vi "LOAD CELL READ.vi"(8 "error in (no error)":errorcluster, 11 "main ref":T1) -> (0 "error out":errorcluster)   [LabVIEW 2025]
uses:
  controls/LAB-IQ UI Data.ctl
  Traction Loop/Traction Receipe Enum.ctl
  <vilib>/Analysis/baseanly.llb/Mean (DBL).vi
  <vilib>/Analysis/5stat.llb/RMS (DBL).vi
  <vilib>/Analysis/NI_AALBase.lvlib
  <vilib>/ptbypt/NI_PtbyPt.lvlib
  <vilib>/Analysis/NI_AALPro.lvlib
  <vilib>/Analysis/Matrix/NI_Matrix.lvlib
  <vilib>/Analysis/Matrix/Numeric/Conversions/Matrix To Array - RM.vi
  <vilib>/Analysis/Matrix/Numeric/Conversions/Array To Matrix - RA.vi
panel:
  out "Fload 3":dbl
  out "Fload 2":dbl
  out "Fload":dbl
  out "Friction":dbl
  out "Load Temp":dbl
  out "Zload":dbl
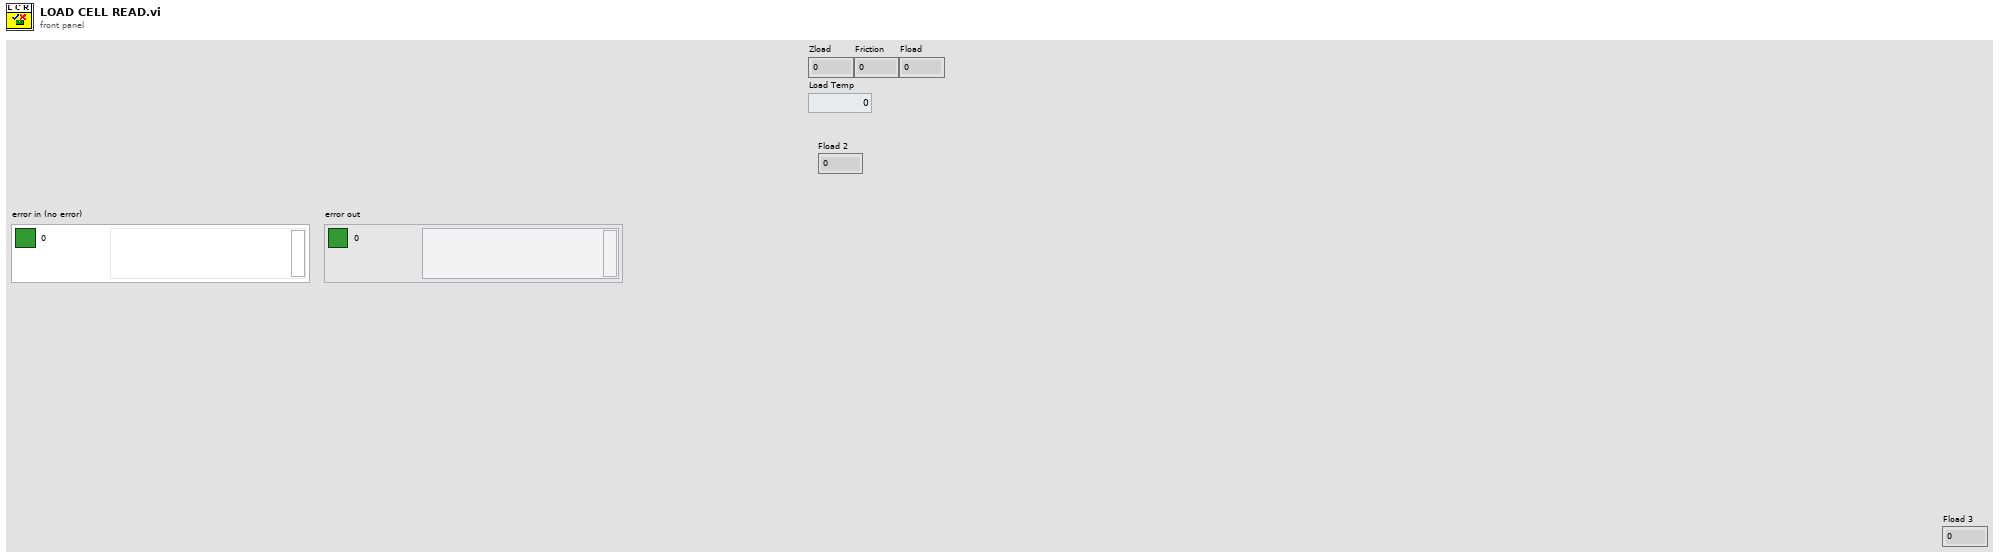
[diagram p1: front panel]
types:
  T1 = typedef "LAB-IQ UI Data.ctl" = cluster{"Main Home Screen":cluster{"GUI":refnum<vi>, "Platform Settings":refnum<vi>, "Configure":refnum<vi>, "Home":refnum<vi>, "EXIT":refnum<vi>, "service 2":refnum<vi>, "MainPage":refnum<vi>, "Analysis":refnum<vi>}, "Platform Settings":cluster{"mm/s  Surge":refnum<vi>, "Update Surge Speed":refnum<vi>, "Drive Error":refnum<vi>, "Disable Axis Jog Soft Limits":refnum<vi>, "mm/s  Sway":refnum<vi>, "Sway and Surge COM Status":refnum<vi>, "Heave COM Status":refnum<vi>, "Enable Platform":refnum<vi>, "Surge Forward Main":refnum<vi>, "Sway Right Main":refnum<vi>, "Sway Left Main":refnum<vi>, "Heave Down Main":refnum<vi>, "Heave Up main":refnum<vi>, "Update Sway Speed":refnum<vi>, "Update Heave Speed":refnum<vi>, "mm/s Heave":refnum<vi>, "mm/sec":refnum<vi>, "mm":refnum<vi>, "Surge Backward Main":refnum<vi>}, "Analysis Screen":cluster{"Analysis Home":refnum<vi>, "Surface Analysis":refnum<vi>, "Imaging":refnum<vi>, "Image Analysis":refnum<vi>, "Post Analysis":refnum<vi>}, "Config Screen":cluster{"Select Load Head":refnum<vi>, "Notes :":refnum<vi>, "FILE":refnum<vi>, "Sample ID :":refnum<vi>, "Operator ID :":refnum<vi>, "Operator Name :":refnum<vi>, "Auto":refnum<vi>}, "Motion Module":cluster{"zNL":refnum<vi>, "NL disp":refnum<vi>, "Rotary Tab":refnum<vi>, "Motion Direction:  3":refnum<vi>, "E.Velocity 2":refnum<vi>, "e.v/ssr 2":refnum<vi>, "Enter Fixed E.Velocity 2":refnum<vi>, "Enter Final SRR 2":refnum<vi>, "Enter initial SRR 2":refnum<vi>, "Enter Fixed SRR 2":refnum<vi>, "Enter the Final E.Velocity (m/s) 2":refnum<vi>, "Enter initial E.Velocity (m/s) 2":refnum<vi>, "Final Speed (RPM) 3":refnum<vi>, "Initial Speed (RPM) 2":refnum<vi>, "Enter the Final Velocity (m/s) 3":refnum<vi>, "Enter initial Velocity (m/s)  3":refnum<vi>, "Ramp Up 2":refnum<vi>, "TEST SELECTION":refnum<vi>, "SPEED SELECTION : ":refnum<vi>, "Angular Oscillation Set":refnum<vi>, "Traction":refnum<vi>, "Step Speed":refnum<vi>, "StepTable For Load-Speed":refnum<vi>, "StepTable For Speed":refnum<vi>, "Surge Forward MM":refnum<vi>, "Surge Backward MM":refnum<vi>, "M3 Image":refnum<vi>, "String 39":refnum<vi>, "Sway Left MM":refnum<vi>, "Sway Right MM":refnum<vi>, "Disable Axis Jog Soft Limits":refnum<vi>, "mm":refnum<vi>, "Heave Down MM":refnum<vi>, "Heave Up MM":refnum<vi>, "Wear Track Diameter (mm)":refnum<vi>, "Set WTD":refnum<vi>, "HomeScratch":refnum<vi>, "HomeRot":refnum<vi>, "PlaceModule":refnum<vi>, "Enter the Angle (Deg)":refnum<vi>, "Enter the Frequency (Hz)":refnum<vi>, "Motion Mode:":refnum<vi>, "LR Sway":refnum<vi>, "Rot Hor":refnum<vi>, "Scratch":refnum<vi>, "LR Cam":refnum<vi>, "MMBack":refnum<vi>, "MMNext":refnum<vi>, "Rot Ver":refnum<vi>, "Rotary Module Selection":refnum<vi>, "calculate rotary":refnum<vi>, "SPEED SELECTION : rotary":refnum<vi>, "Import 2":refnum<vi>, "Save 2":refnum<vi>, "File Path :  2":refnum<vi>, "String 45":refnum<vi>, "StepTable For Speed 3":refnum<vi>, "Enter the Speed(mm/sec)":refnum<vi>, "Enter the Speed(RPM)":refnum<vi>, "Enter Scratch Speed (mm/s):":refnum<vi>, "SwaySpeed Set":refnum<vi>, "Scartch Offset":refnum<vi>, "Motion type:":refnum<vi>, "HomeScratch 2":refnum<vi>, "Enter Scratch length (mm):":refnum<vi>, "Wear Track Diameter":refnum<vi>, "Rotary Speed Exced":refnum<vi>, "Scratch Mode":refnum<vi>, "No of Scratch":refnum<vi>}, "Environmental control":cluster{"Humidity  Status  3":refnum<vi>, "Low Temp  Status  2":refnum<vi>, "TK4 status 2":refnum<vi>, "Stage Temperature":refnum<vi>, "Sample Temperature":refnum<vi>, "Humidity (Amb)":refnum<vi>, "Clear List":refnum<vi>, "Add to list":refnum<vi>, "Wear":refnum<vi>, "Vibration":refnum<vi>, "Humidity (Chamber)":refnum<vi>, "Temperature (Chamber)":refnum<vi>, "ECR ":refnum<vi>, "Temperature (Amb)":refnum<vi>, "Microphone":refnum<vi>, "Acoustic Emission 3":refnum<vi>, "SNext":refnum<vi>, "APBack":refnum<vi>, "Enter the Temperature (°C):":refnum<vi>, "Enter the Stage \nTemperature (°C):":refnum<vi>, "Enter the Humidity (%Rh):":refnum<vi>, "Low Temp":refnum<vi>, "High Temp":refnum<vi>, "Humidity":refnum<vi>, "Sensors Picked":refnum<vi>}, "About Screen":cluster{"Password":refnum<vi>, "Home Service":refnum<vi>, "Advanced Setting":refnum<vi>, "About Tab":refnum<vi>, "ECR Port:":refnum<vi>, "Ramp Port:":refnum<vi>, "Installation/Replacement completed":refnum<vi>, "Loahead":refnum<vi>, "Heave and Surge COM Port:":refnum<vi>, "Sway COM Port:":refnum<vi>, "Temp Modbus:":refnum<vi>, "Humidity Port:":refnum<vi>, "Edit Gain Constants":refnum<vi>, "Save Gain Constants":refnum<vi>}, "Main Screen":cluster{"Main Screen Tab":refnum<vi>, "Angle and Frequency":refnum<vi>, "Stroke (mm)":refnum<vi>, "Angle (Deg)":refnum<vi>, "Main Speed Tab":refnum<vi>, "MTM MOTOR DISPLAY":refnum<vi>, "Disc Speed (m/sec)":refnum<vi>, "Ball Speed (m/sec)":refnum<vi>, "Disc Speed (RPM)":refnum<vi>, "Ball Speed (RPM)":refnum<vi>, "SPEED TAB":refnum<vi>, "Speed (m/sec)":refnum<vi>, "Set Speed (m/sec)":refnum<vi>, "Speed (RPM)":refnum<vi>, "Set Speed":refnum<vi>, "Time Tab":refnum<vi>, "Time ( HH:MM:SS ) 2":refnum<vi>, "Test Duration":refnum<vi>, "Test Duration 4":refnum<vi>, "TEST CYCLE":refnum<vi>, "TOTAL CYCLES":refnum<vi>, "Set Load (N)":refnum<vi>, "Temp Tabs":refnum<vi>, "Heater":refnum<vi>, "TK4 status":refnum<vi>, "ChamberTemp":refnum<vi>, "SetTmp":refnum<vi>, "Controller  Status":refnum<vi>, "ChamberTemp 2":refnum<vi>, "SetTmp 2":refnum<vi>, "Controller  Status 2":refnum<vi>, "ChamberTemp 3":refnum<vi>, "SetTmp 3":refnum<vi>, "Cooling":refnum<vi>, "Load Communication":refnum<vi>, "Ambient \nTemperature":refnum<vi>, "HumCOMStatus":refnum<vi>, "Ambient\n Humidity":refnum<vi>, "Freq (Hz)":refnum<vi>, "Load En":refnum<vi>, "NLt":refnum<vi>, "zNL 2":refnum<vi>, "Humidity On":refnum<vi>, "humidity disp":refnum<vi>, "Set Humidity":refnum<vi>, "NL disp 2":refnum<vi>, "Humidity On 2":refnum<vi>, "humidity disp 2":refnum<vi>, "Set Humidity 2":refnum<vi>, "NL disp 3":refnum<vi>, "AppLoadSeq scratch":refnum<vi>, "Stop Scratch":refnum<vi>, "ClrLog":refnum<vi>, "Trip Log":refnum<vi>, "STOP":refnum<vi>, "Start Test":refnum<vi>, "Test status":refnum<vi>, "AR Led":refnum<vi>, "Data":refnum<vi>, "Health":refnum<vi>, "Sway COM Status":refnum<vi>, "Heave COM Status":refnum<vi>, "Grp Tab":refnum<vi>, "Sub Graph":refnum<vi>, "SD (mm)":refnum<vi>, "Siliding distance Reset Graph":refnum<vi>, "SDGp":refnum<vi>, "Humidity Reset Graph":refnum<vi>, "HumrGp":refnum<vi>, "Acoustic Emission (mV)":refnum<vi>, "Aqucostic Reset Graph":refnum<vi>, "gACQUOS":refnum<vi>, "ECR RESET":refnum<vi>, "ECR":refnum<vi>, "Temperature Reset":refnum<vi>, "Acoustic Emission (mV) 2":refnum<vi>, "Aqucostic Reset Graph 2":refnum<vi>, "gACQUOS 2":refnum<vi>, "ECR RESET 2":refnum<vi>, "ECR 2":refnum<vi>, "Temperature Reset 2":refnum<vi>, "Temperature (deg c)":refnum<vi>, "Speed Reset Graph":refnum<vi>, "Speed Tab":refnum<vi>, "MTM DISC  SPEED":refnum<vi>, "MTM BALL SPEED":refnum<vi>, "speed mm/sec":refnum<vi>, "Hymidity":refnum<vi>, "Humidity Disable trip":refnum<vi>, "CoF Trip  2":refnum<vi>, "Depth Trip":refnum<vi>, "Weart Deapth":refnum<vi>, "Depth Reset Graph":refnum<vi>, "Weart":refnum<vi>, "Depthz":refnum<vi>, "Depth (µm)":refnum<vi>, "WearGp":refnum<vi>, "NL Trip 2":refnum<vi>, "Load pid":refnum<vi>, "Load Disable Trip":refnum<vi>, "Load Reset Graph":refnum<vi>, "NL Display 4":refnum<vi>, "Main Chart 3":refnum<vi>, "BACK":refnum<vi>, "Depth Trip 2":refnum<vi>, "COF TRIP ":refnum<vi>, "Friction Force (N)":refnum<vi>, "FF Reset Graph":refnum<vi>, "FF Disable Trip":refnum<vi>, "FF TRIP":refnum<vi>, "COF Disable Trip":refnum<vi>, "COF Reset Graph":refnum<vi>, "Start Test Temp":refnum<vi>, "zFF":refnum<vi>, "Friction Force (N) Graph":refnum<vi>, "Coefficient of Friction":refnum<vi>, "Scratch Start Test":refnum<vi>, "FF Tab":refnum<vi>, "Cyclic Friction Force (N)":refnum<vi>, "CZ FF":refnum<vi>, "Cyclic Friction Force (N) Graph":refnum<vi>, "Cyclic Coefficient of Friction":refnum<vi>, "Cyclic FF TRIP":refnum<vi>, "Cyclic FF Disable Trip":refnum<vi>, "cyclic COF Disable Trip":refnum<vi>, "cyclic COF TRIP":refnum<vi>, "cyclic COF Reset Graph":refnum<vi>, "Cyclic FF Reset Graph":refnum<vi>, "Test Trip":refnum<vi>, "Multi Scratch Pass":refnum<vi>, "Scratch Start Recording":refnum<vi>}, "Loading":cluster{"Indentation":refnum<vi>, "Reference Sample":refnum<vi>, "Load Cell Communication Slide":refnum<vi>, "com 3":refnum<vi>, "com":refnum<vi>, "DecaForce COM Status":refnum<vi>, "Update":refnum<vi>, "Clear 3":refnum<vi>, "seq":refnum<vi>, "Stribeck table":refnum<vi>, "Stribeck Table  For loading":refnum<vi>, "Loading Mode":refnum<vi>, "Enter the Final Load (N)":refnum<vi>, "Enter the CoF Trip":refnum<vi>, "Enter the Friction Force Trip":refnum<vi>, "Enter the Normal load Trip":refnum<vi>, "Enter the Load  (N)":refnum<vi>, "KiloForce":refnum<vi>, "DecaForce ":refnum<vi>, "MicroForce":refnum<vi>, "LHBack":refnum<vi>, "LHNext":refnum<vi>, "Enter the Loading Rate (N/min)":refnum<vi>, "Message":refnum<vi>, "Warning 2":refnum<vi>, "SSP 0.75":refnum<vi>, "SSP 0.5":refnum<vi>, "SSP 0.3":refnum<vi>, "Warning":refnum<vi>, "gui GIF":refnum<vi>, "Communication is established":refnum<vi>, "AppLoad 4":refnum<vi>, "Multipoint":refnum<vi>, "Load Selection":refnum<vi>}, "PID":cluster{"Ramp MulFac":refnum<vi>, "pulses LoadDiffRamp(2..10)":refnum<vi>, "PulseControlRamp(diff<=3N)":refnum<vi>, "SetLoadDeadband(%) Load(0-10N)":refnum<vi>, "PID gains out delay (microForce)":refnum<vi>, "Ramp":refnum<vi>, "Gain 2":refnum<vi>, "pulses LoadDiff(2..10)":refnum<vi>, "pulses LoadDiff(11..50)":refnum<vi>, "PulseControl(diff<=3N)":refnum<vi>, "SetLoadDeadband(%)  2":refnum<vi>, "Dummy Run":refnum<vi>, "Vertical load (N)":refnum<vi>, "AutoTune":refnum<vi>, "Offset 3 ":refnum<vi>, "apply load":refnum<vi>, "Offset  3":refnum<vi>, "apply load 2":refnum<vi>, "Enter ByPass Load":refnum<vi>, "reinit 3":refnum<vi>, "output range delay":refnum<vi>, "PID gains out delay":refnum<vi>, "Bypass Load":refnum<vi>, "pulsesSent":refnum<vi>, "pulses ":refnum<vi>, "actpid":refnum<vi>, "gFF Rot":refnum<vi>, "pulses LoadDiff(21..1000)":refnum<vi>, "Delay":refnum<vi>, "deadband":refnum<vi>}, "Config Parameters":cluster{"Tab Control 3":refnum<vi>, "Tab Control 19":refnum<vi>, "SAMPLES":refnum<vi>, "Re-initilaize":refnum<vi>, "Filter ON/OFF":refnum<vi>, "TracHomeSurgeOffsetCounts 10MM":refnum<vi>, "TracHomeSwayOffsetCounts 10MM":refnum<vi>, "Acoustic Emission:":refnum<vi>, "Apply Filter (FF)":refnum<vi>, "Filter% 2":refnum<vi>, "Apply Filter (Load)":refnum<vi>, "Filter% ":refnum<vi>, "Sway distance (mm)":refnum<vi>, "Surge distance (mm)":refnum<vi>, "DataSavingLoopDelay(ms)":refnum<vi>, "SAVE 2":refnum<vi>, "Enter Distance":refnum<vi>, "Sway Counts:":refnum<vi>, "Distance (mm): 3":refnum<vi>, "Surge Counts:":refnum<vi>, "Distance (mm): 2":refnum<vi>, "Distance (mm):":refnum<vi>, "Heave Counts:":refnum<vi>, "LRMHomeSurgeOffsetCounts":refnum<vi>, "LRMHomeSwayOffsetCounts":refnum<vi>, "TracHomeSurgeOffsetCounts 20MM":refnum<vi>, "TracHomeSwayOffsetCounts 20MM":refnum<vi>, "RotHomeSwayOffsetCounts":refnum<vi>, "RotHomeSurgeOffsetCounts":refnum<vi>, "Heave distance":refnum<vi>, "Zmm":refnum<vi>, "Heave Pulses/mm":refnum<vi>, "Surge Pulses/mm":refnum<vi>, "Sway Pulses/mm":refnum<vi>, "Heave Pitch":refnum<vi>, "Surge Pitch":refnum<vi>, "Sway Pitch":refnum<vi>, "Heave PPR":refnum<vi>, "Surge PPR":refnum<vi>, "Sway PPR":refnum<vi>, "Tab Control 5":refnum<vi>, "Tab Control 14":refnum<vi>, "Tab Control 26":refnum<vi>, "AE":refnum<vi>, "Heave Loop Delay":refnum<vi>, "Heave PID Speed":refnum<vi>, "Surge Jog Speed":refnum<vi>, "Heave Jog Speed":refnum<vi>, "Sway Loop Delay":refnum<vi>, "Sway PID Speed":refnum<vi>, "Sway Jog Speed":refnum<vi>, "DEPTH TRIP VALUE":refnum<vi>, "LOAD TRIP VALUE":refnum<vi>, "DEPTH TRIP   ENABLE":refnum<vi>, "LOAD TRIP  ENABLE":refnum<vi>, "CYCLIC FF TRIP VALUE":refnum<vi>, "FF TRIP VALUE":refnum<vi>, "CYCLIC CoF TRIP VALUE":refnum<vi>, "COF TRIP VALUE":refnum<vi>, "CYCLIC COF TRIP  ENABLE":refnum<vi>, "CYCLIC FF TRIP  ENABLE":refnum<vi>, "FF TRIP  ENABLE":refnum<vi>, "COF TRIP  ENABLE":refnum<vi>, "JOG TRIP LOAD VALUE (N)":refnum<vi>, "Rotary Vertical":refnum<vi>, "Traction":refnum<vi>, "Scratch":refnum<vi>, "LRM CAM":refnum<vi>, "Sway LRM":refnum<vi>, "Rotary Horizontal":refnum<vi>}, "Loading Com Port":cluster{"ClearAll":refnum<vi>, "Mz(Nm)":refnum<vi>, "My(Nm)":refnum<vi>, "Mx(Nm)":refnum<vi>, "Save Dwell":refnum<vi>, "Acq Delay (ms)":refnum<vi>, "Burst Delay (ms)":refnum<vi>, "model":refnum<vi>, "SN":refnum<vi>, "FFx(N)":refnum<vi>, "Sensor IP":refnum<vi>, "Port":refnum<vi>, "FFy(N)":refnum<vi>, "Load(N)":refnum<vi>, "delete Handle":refnum<vi>, "Create Handle":refnum<vi>, "ft_data":refnum<vi>, "ft_range":refnum<vi>, "ft_data 2":refnum<vi>, "stop 6":refnum<vi>, "running_flag":refnum<vi>, "ft_udp_handle":refnum<vi>, "get-data-return":refnum<vi>, "get-range-return":refnum<vi>, "zero-return":refnum<vi>, "filter-return":refnum<vi>, "initial-return":refnum<vi>, "deleteHandle-result":refnum<vi>, "Load Cell Temp":refnum<vi>, "Load Cell":refnum<vi>, "ZeroAll":refnum<vi>, "FORCE (N)":refnum<vi>, "TORQUE (N-m)":refnum<vi>}, "Heave AND Surge":cluster{"SURGE POSE":refnum<vi>, "error out Read":refnum<vi>, "HEAVE POSE":refnum<vi>, "State":refnum<vi>, "Homed":refnum<vi>, "Sequence ID":refnum<vi>, "error out Write":refnum<vi>, "faultCode":refnum<vi>, "Ack ID":refnum<vi>, "SPEED":refnum<vi>, "Distance":refnum<vi>, "Mode Command":refnum<vi>, "Heave and Surge Read":refnum<vi>, "Read Heave Temp":refnum<vi>, "Spare 15":refnum<vi>, "Spare 14":refnum<vi>, "Spare 13":refnum<vi>, "Spare 12":refnum<vi>, "Spare 11":refnum<vi>, "Spare 10":refnum<vi>, "Spare 9":refnum<vi>, "Spare 8":refnum<vi>, "Spare 7":refnum<vi>, "Spare 6":refnum<vi>, "Spare 5":refnum<vi>, "Spare 4":refnum<vi>, "Spare 2":refnum<vi>, "Spare 1":refnum<vi>, "Node Id":refnum<vi>, "Spare 3":refnum<vi>, "SPARE 4":refnum<vi>, "SPARE 3":refnum<vi>, "SPARE 2":refnum<vi>, "SPARE 1":refnum<vi>, "fwMajor":refnum<vi>, "fwMinor":refnum<vi>, "Manual Write":refnum<vi>, "Heave and Surge Write":refnum<vi>, "SPARE 5":refnum<vi>, "Reserved ":refnum<vi>, "SPARE 8":refnum<vi>, "SPARE 6":refnum<vi>, "SPARE 7":refnum<vi>, "SPARE 17":refnum<vi>, "SPARE 16":refnum<vi>, "SPARE 15":refnum<vi>, "SPARE 14":refnum<vi>, "SPARE 13":refnum<vi>, "SPARE 12":refnum<vi>, "SPARE 11":refnum<vi>, "SPARE 10":refnum<vi>, "SPARE 9":refnum<vi>, "System UPTIME":refnum<vi>, "Missed Packets":refnum<vi>, "faultCode Surge Right":refnum<vi>, "faultCode Surge Left":refnum<vi>, "faultCode Heave":refnum<vi>, "UPLINK HEAVE":refnum<vi>, "DOWNLINK HEAVE":refnum<vi>}, "New PID LOGIC":cluster{"Fine Tune Zone":refnum<vi>, "PID SDelay":refnum<vi>, "Max_pos_limit":refnum<vi>, "Min_pos_limit":refnum<vi>, "i_limit":refnum<vi>, "pct_scale":refnum<vi>, "Deadband":refnum<vi>, "Kd":refnum<vi>, "Ki":refnum<vi>, "Kp":refnum<vi>, "Current Position":refnum<vi>, "Set Load":refnum<vi>, "Current Load":refnum<vi>, "Pulse delta":refnum<vi>, "Init Step":refnum<vi>, "Max Step Linit":refnum<vi>, "min_deadband_floor":refnum<vi>, "dynamic_spindle_noise_scalar":refnum<vi>, "min_finetune_floor":refnum<vi>, "filter_alpha":refnum<vi>, "PID":refnum<vi>}, "SWAY ":cluster{"fwMajor":refnum<vi>, "Homed":refnum<vi>, "Rotary POSE":refnum<vi>, "State":refnum<vi>, "SWAY POSE":refnum<vi>, "Ack ID":refnum<vi>, "faultCode":refnum<vi>, "Node Id":refnum<vi>, "fwMinor":refnum<vi>, "Spare 6":refnum<vi>, "Spare 5":refnum<vi>, "Spare 4":refnum<vi>, "Spare 3":refnum<vi>, "Spare 2":refnum<vi>, "Spare 1":refnum<vi>, "Spare 7":refnum<vi>, "SPARE  5":refnum<vi>, "error out Write  SWAY ":refnum<vi>, "error out Read SWAY ":refnum<vi>, "Manual Write SWAY ":refnum<vi>, "SWAY WRITE":refnum<vi>, "SPARE  4":refnum<vi>, "SPARE  3":refnum<vi>, "SPARE 2":refnum<vi>, "SPARE 1":refnum<vi>, "Spare 15":refnum<vi>, "Spare 14":refnum<vi>, "Spare 13":refnum<vi>, "Spare 12":refnum<vi>, "Spare 11":refnum<vi>, "Spare 9":refnum<vi>, "Spare 8":refnum<vi>, "SPEED":refnum<vi>, "Distance":refnum<vi>, "Mode Command":refnum<vi>, "Sequence ID":refnum<vi>, "SWAY READ":refnum<vi>, "Spare 10":refnum<vi>, "Read SWAY Temp":refnum<vi>, "faultCode Sway ":refnum<vi>, "Missed Packets":refnum<vi>, "System UPTIME sway":refnum<vi>, "SPARE 6":refnum<vi>, "SPARE 7":refnum<vi>, "SPARE 9":refnum<vi>, "SPARE 11":refnum<vi>, "SPARE 10":refnum<vi>, "SPARE 8":refnum<vi>, "SPARE 13":refnum<vi>, "SPARE 12":refnum<vi>, "SPARE 17":refnum<vi>, "SPARE 16":refnum<vi>, "SPARE 15":refnum<vi>, "SPARE 14":refnum<vi>, "Reserved":refnum<vi>, "faultCode Rotary":refnum<vi>, "UPLINK SWAY":refnum<vi>, "DOWNLINK SWAY":refnum<vi>}, "Analysis Screen":cluster{"Analysis Home":refnum<vi>, "Refresh 2":refnum<vi>, "MEAN 4":refnum<vi>, "SD 4":refnum<vi>, "VARIANCE 4":refnum<vi>, "MEAN  3":refnum<vi>, "SD  3":refnum<vi>, "VARIANCE  3":refnum<vi>, "MEAN 2":refnum<vi>, "SD  2":refnum<vi>, "VARIANCE 2":refnum<vi>, "MEAN":refnum<vi>, "SD":refnum<vi>, "VARIANCE":refnum<vi>, "File 4 Discription":refnum<vi>, "OPEN 4":refnum<vi>, "File Name 4":refnum<vi>, "OPEN 3":refnum<vi>, "File 3 Discription":refnum<vi>, "File Name 3":refnum<vi>, "Y-AXIS":refnum<vi>, "X-AXIS":refnum<vi>, "XY Graph":refnum<vi>, "File Name 2":refnum<vi>, "File Name 1":refnum<vi>, "OPEN 2":refnum<vi>, "OPEN 1":refnum<vi>, "File 1 Discription ":refnum<vi>, "File 2 Discription":refnum<vi>, "Export":refnum<vi>, "File Format":refnum<vi>}, "Traction":cluster{"faultCode Traction 2":refnum<vi>, "faultCode Traction 1":refnum<vi>, "Missed Packets":refnum<vi>, "System UPTIME Traction":refnum<vi>, "SPARE 17":refnum<vi>, "SPARE 16":refnum<vi>, "SPARE 15":refnum<vi>, "SPARE 14":refnum<vi>, "SPARE 13":refnum<vi>, "SPARE 12":refnum<vi>, "SPARE 11":refnum<vi>, "SPARE 10":refnum<vi>, "SPARE 9":refnum<vi>, "SPARE 8":refnum<vi>, "SPARE 7":refnum<vi>, "SPARE 6":refnum<vi>, "Reserved":refnum<vi>, "SPARE  5":refnum<vi>, "Manual Write TRACTION":refnum<vi>, "TRACTION WRITE":refnum<vi>, "SPARE  4":refnum<vi>, "SPARE  3":refnum<vi>, "SPARE 2":refnum<vi>, "SPARE 1":refnum<vi>, "Spare 7":refnum<vi>, "Spare 6":refnum<vi>, "Spare 5":refnum<vi>, "Spare 4":refnum<vi>, "Spare 2":refnum<vi>, "Spare 1":refnum<vi>, "Node Id":refnum<vi>, "Read TRACTION Temp":refnum<vi>, "fwMinor":refnum<vi>, "fwMajor":refnum<vi>, "faultCode":refnum<vi>, "TRACTION POSE":refnum<vi>, "TRACTION POSE 2":refnum<vi>, "Homed":refnum<vi>, "State":refnum<vi>, "Ack ID":refnum<vi>, "SPEED":refnum<vi>, "Distance":refnum<vi>, "Mode Command":refnum<vi>, "Sequence ID":refnum<vi>, "error out Read TRACTION":refnum<vi>, "error out Write  TRACTION":refnum<vi>, "TRACTION READ":refnum<vi>, "Spare 3":refnum<vi>, "Downlink traction":refnum<vi>, "Uplink Traction":refnum<vi>}, "Traction reciepe":cluster{"SRR Sweep Range (%) Stribeck":refnum<vi>, "Traction Receipe":refnum<vi>, "Total Execution Time":refnum<vi>, "Total Steps":refnum<vi>, "Duration / Step (s)  Stribeck":refnum<vi>, "STRIBECK Fixed SRR List (%)":refnum<vi>, "Duration / Step (s) Traction":refnum<vi>, "SRR Sweep Range (%) traction":refnum<vi>, "Rolling Speed (mm/s)":refnum<vi>, "Temperature Stages (°C)":refnum<vi>, "Ball Load (N)":refnum<vi>, "Lubricant Name":refnum<vi>, "Profile File Name":refnum<vi>, "SET entrainment Velocity":refnum<vi>, "Test Array Size":refnum<vi>, "SRR INDEX [ STRIBECK]":refnum<vi>, "Stribeck Size":refnum<vi>, "SET SRR":refnum<vi>, "ELAPSED TIMER ":refnum<vi>, "BALL SET RPM":refnum<vi>, "DISC SET RPM":refnum<vi>, "SET LOAD":refnum<vi>, "TEMPERATURE READ":refnum<vi>, "SET TEMPERATURE":refnum<vi>, "Traction Size":refnum<vi>, "DISC SPEED (rpm)":refnum<vi>, "BALL SPEED (rpm)":refnum<vi>, "BALL WEAR TRACK":refnum<vi>, "DISC WEARTRACK":refnum<vi>, "SRR INDEX [ TRACTION]":refnum<vi>, "Start Index Type":refnum<vi>, "Enum - Menu":refnum<vi>, "Ball (mm/sec)":refnum<vi>, "Disc (mm/sec)":refnum<vi>}, "Traction Control":cluster{"HomeTraction":refnum<vi>, "Demo Mode Display":refnum<vi>, "Traction Message":refnum<vi>, "Traction Step Update Details":refnum<vi>, "Main Tab sequence for selection":refnum<vi>, "Ramp Tab":refnum<vi>, "e.v/ssr":refnum<vi>, "Enter Fixed E.Velocity":refnum<vi>, "Enter Final SRR":refnum<vi>, "Enter initial SRR":refnum<vi>, "Enter Fixed SRR":refnum<vi>, "Enter the Final E.Velocity (m/s)":refnum<vi>, "Enter initial E.Velocity (m/s)":refnum<vi>, "Ball WTD":refnum<vi>, "E.Velocity":refnum<vi>, "Enter the Final Velocity (m/s)":refnum<vi>, "Enter initial Velocity (m/s)":refnum<vi>, "Ramp Up   Disc":refnum<vi>, "Initial DiscSpeed (RPM)":refnum<vi>, "Final Speed (RPM) Ball":refnum<vi>, "Final Speed (RPM)":refnum<vi>, "Initial Speed (RPM) Ball":refnum<vi>, "Enter the Final Velocity (m/s) Ball":refnum<vi>, "Enter initial Velocity (m/s) Ball":refnum<vi>, "Ramp Up":refnum<vi>, "ExceedBallSpeed step":refnum<vi>, "ExceedDiscSpeed":refnum<vi>, "BallSpeed Exceed Indication":refnum<vi>, "Apply":refnum<vi>, "SPEED SELECTION : MTM":refnum<vi>, "SPEED SELECTION : MTM 2":refnum<vi>, "TEST SELECTION (MTM)":refnum<vi>, "MTM Test Selection":refnum<vi>, "File Path Tab":refnum<vi>, "File Path String":refnum<vi>, "Save":refnum<vi>, "Save  2":refnum<vi>, "Import ":refnum<vi>, "File Path :":refnum<vi>, "Step Sequence Indication Tab":refnum<vi>, "Step Sequence Indication":refnum<vi>, "Calculate Step":refnum<vi>, "StepTable":refnum<vi>, "ExceedDiscSpeed  Cinstant Speed":refnum<vi>, "ExceedBallSpeed Constant":refnum<vi>, "TEST SELECTION (MTM) 2":refnum<vi>, "SPEED SELECTION : MTM 3":refnum<vi>, "MTM Test Selection 2":refnum<vi>, "Enter the Speed (m/sec): ":refnum<vi>, "Enter the Speed (m/sec):  2":refnum<vi>, "Enter the Speed (RPM):":refnum<vi>, "Lower Spped ":refnum<vi>, "Upper":refnum<vi>, "Enter the Speed (RPM):Ball":refnum<vi>, "Disc Motion Direction: ":refnum<vi>, "Ball Motion Direction :":refnum<vi>, "Motion Mode: ":refnum<vi>, "Wear Track Diameter (mm) ":refnum<vi>, "Disc Speed Indicator":refnum<vi>, "ExceedBallSpeed":refnum<vi>}, "Acquostic":cluster{"Last Config Rejected ":refnum<vi>, "rx command count":refnum<vi>, "Current Filter Id":refnum<vi>, "Isolated Gain":refnum<vi>, "DAQ Status":refnum<vi>, "error out":refnum<vi>, "error in (no error)":refnum<vi>, "Uplink Packet":refnum<vi>, "data out":refnum<vi>, "Downlink Packet":refnum<vi>, "Signal Energy":refnum<vi>, "Amplitude db_AE":refnum<vi>, "Peak Amplitude":refnum<vi>, "AE Ring-Down Counts":refnum<vi>, "Gains":refnum<vi>, "Manual Write Acquostic":refnum<vi>}}
  T2 = enum16{"INIT", "SETLOWPASSFILTER", "SETZERO", "GETSENSORINFO", "GETRANGE", "ZEROALL", "READDATA", "UNINITIAL", "DELETEHANDLE"}
  T3 = typedef "NI_Matrix.lvlib/RealMatrix.ctl" = dbl[][]
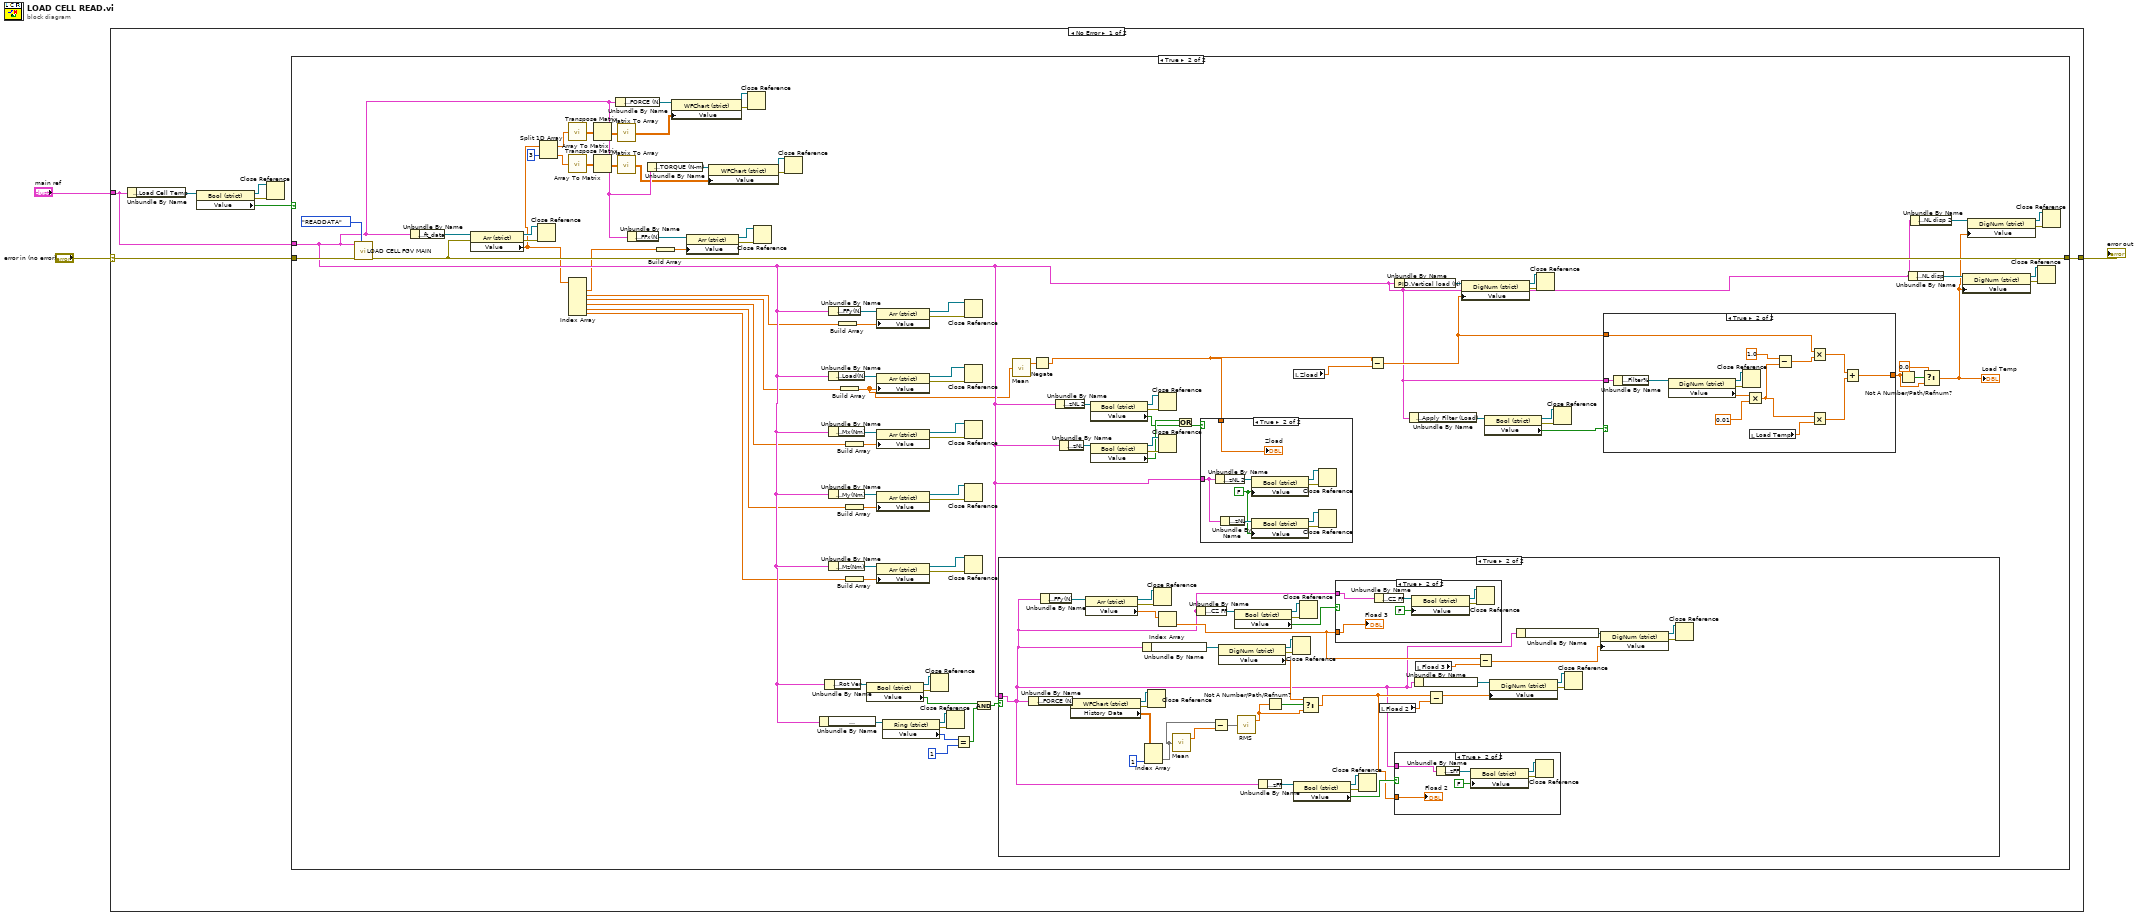
[diagram p0: block diagram]
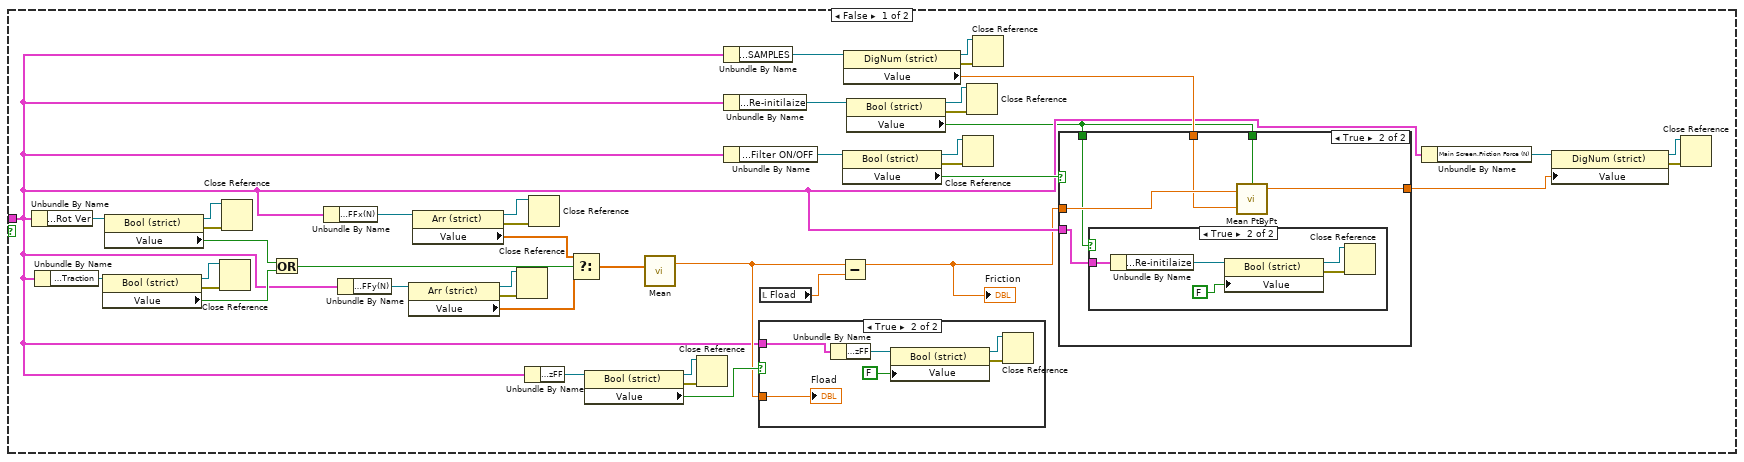
[diagram p3: hidden frame]
diagram:
  n1 = case shown="No Error" "error in (no error)" {
    selector: "error in (no error)" -> [w6 _]
    tunnel: "main ref" -> [w4 _]
    tunnel: [w5 _] -> w1
    frame No Error {
      n2 = Unbundle By Name(w4) -> ("Loading Com Port.Load Cell Temp"=w8:refnum<vi>)
      n3 = property class="Bool (strict)"(reference=w8) -> (reference out=w10:refnum<vi>, error out=w9:errorcluster, "Value"=w7:bool)  [unwired: 1 in]
      n4 = Close Reference(reference=w10, error in (no error)=w9) -> ()  [unwired: 1 out]
      n5 = case shown="True" w7 {
        tunnel: w6 -> [w11 w105]
        tunnel: [w11 w101] -> w5
        tunnel: w4 -> [_ w26]
        frame False {
        }
        frame True {
          n6 = call "LOAD CELL FGV MAIN.vi"("Enum"=T2."READDATA", "error in (no error)"=w105, "main ref"=w26) -> ("error IO"=w101:errorcluster)  [unwired: 8 in]
          n7 = Unbundle By Name(w26) -> ("Loading Com Port.ft_data"=w103:refnum<vi>)
          n8 = property class="Arr (strict)"(reference=w103, error in=w101) -> (reference out=w100:refnum<vi>, error out=w102:errorcluster, "Value"=w24:dbl[])
          n9 = Close Reference(reference=w100, error in (no error)=w102) -> ()  [unwired: 1 out]
          n10 = Split 1D Array(array=w24, index=3) -> (first subarray=w34:dbl[], second subarray=w31:dbl[])
          n11 = call-poly <vilib>:"Array To Matrix.vi"("Real 1D Array"=w34) -> ("Real Matrix (Column Vector)"=w36:T3)
          n12 = call-poly <vilib>:"Array To Matrix.vi"("Real 1D Array"=w31) -> ("Real Matrix (Column Vector)"=w33:T3)
          n13 = Index Array(array=w24) -> (element #1=w23:dbl, element #2=w21:dbl, element #3=w19:dbl, element #4=w18:dbl, element #5=w15:dbl, element #6=w13:dbl)  [unwired: 6 in]
          n14 = Transpose Matrix(1:w36) -> (0:w35:T3)
          n15 = Transpose Matrix(1:w33) -> (0:w32:T3)
          n16 = Unbundle By Name(w26) -> ("Loading Com Port.FORCE (N)"=w99:refnum<vi>)
          n17 = call-poly <vilib>:"Matrix To Array.vi"("Real Matrix"=w35) -> ("Real 2D Array"=w30:dbl[][])
          n18 = call-poly <vilib>:"Matrix To Array.vi"("Real Matrix"=w32) -> ("Real 2D Array"=w25:dbl[][])
          n19 = Unbundle By Name(w26) -> ("Loading Com Port.FFx(N)"=w94:refnum<vi>)
          n20 = Unbundle By Name(w26) -> ("Loading Com Port.TORQUE (N-m)"=w29:refnum<vi>)
          n21 = Build Array(w23) -> (w22:dbl[])
          n22 = property class="WFChart (strict)"(reference=w99, "Value"=w30) -> (reference out=w97:refnum<vi>, error out=w98:errorcluster)  [unwired: 1 in]
          n23 = property class="Arr (strict)"(reference=w94, "Value"=w22) -> (reference out=w96:refnum<vi>, error out=w95:errorcluster)  [unwired: 1 in]
          n24 = property class="WFChart (strict)"(reference=w29, "Value"=w25) -> (reference out=w27:refnum<vi>, error out=w28:errorcluster)  [unwired: 1 in]
          n25 = Close Reference(reference=w97, error in (no error)=w98) -> ()  [unwired: 1 out]
          n26 = Close Reference(reference=w96, error in (no error)=w95) -> ()  [unwired: 1 out]
          n27 = Close Reference(reference=w27, error in (no error)=w28) -> ()  [unwired: 1 out]
          n28 = Unbundle By Name(w26) -> ("Motion Module.Motion Mode:"=w43:refnum<vi>)
          n29 = Unbundle By Name(w26) -> ("Motion Module.Rot Ver"=w48:refnum<vi>)
          n30 = Unbundle By Name(w26) -> ("Loading Com Port.FFy(N)"=w91:refnum<vi>)
          n31 = Unbundle By Name(w26) -> ("Loading Com Port.Load(N)"=w90:refnum<vi>)
          n32 = Unbundle By Name(w26) -> ("Loading Com Port.Mx(Nm)"=w85:refnum<vi>)
          n33 = Unbundle By Name(w26) -> ("Loading Com Port.My(Nm)"=w84:refnum<vi>)
          n34 = Unbundle By Name(w26) -> ("Loading Com Port.Mz(Nm)"=w79:refnum<vi>)
          n35 = Build Array(w21) -> (w20:dbl[])
          n36 = Build Array(w19) -> (w16:dbl[])
          n37 = Build Array(w18) -> (w17:dbl[])
          n38 = Build Array(w15) -> (w14:dbl[])
          n39 = Build Array(w13) -> (w12:dbl[])
          n40 = property class="Bool (strict)"(reference=w48) -> (reference out=w46:refnum<vi>, error out=w47:errorcluster, "Value"=w40:bool)  [unwired: 1 in]
          n41 = property class="Arr (strict)"(reference=w91, "Value"=w20) -> (reference out=w93:refnum<vi>, error out=w92:errorcluster)  [unwired: 1 in]
          n42 = property class="Arr (strict)"(reference=w90, "Value"=w16) -> (reference out=w88:refnum<vi>, error out=w89:errorcluster)  [unwired: 1 in]
          n43 = property class="Arr (strict)"(reference=w85, "Value"=w17) -> (reference out=w87:refnum<vi>, error out=w86:errorcluster)  [unwired: 1 in]
          n44 = property class="Arr (strict)"(reference=w84, "Value"=w14) -> (reference out=w82:refnum<vi>, error out=w83:errorcluster)  [unwired: 1 in]
          n45 = property class="Arr (strict)"(reference=w79, "Value"=w12) -> (reference out=w81:refnum<vi>, error out=w80:errorcluster)  [unwired: 1 in]
          n46 = property class="Ring (strict)"(reference=w43) -> (reference out=w45:refnum<vi>, error out=w44:errorcluster, "Value"=w42:u16)  [unwired: 1 in]
          n47 = Close Reference(reference=w46, error in (no error)=w47) -> ()  [unwired: 1 out]
          n48 = Close Reference(reference=w45, error in (no error)=w44) -> ()  [unwired: 1 out]
          n49 = Equal?(x=w42, y=u16 1) -> (x = y?=w39:bool)
          n50 = Close Reference(reference=w93, error in (no error)=w92) -> ()  [unwired: 1 out]
          n51 = Close Reference(reference=w88, error in (no error)=w89) -> ()  [unwired: 1 out]
          n52 = Close Reference(reference=w87, error in (no error)=w86) -> ()  [unwired: 1 out]
          n53 = Close Reference(reference=w82, error in (no error)=w83) -> ()  [unwired: 1 out]
          n54 = Close Reference(reference=w81, error in (no error)=w80) -> ()  [unwired: 1 out]
          n55 = And(x=w40, y=w39) -> (x .and. y?=w38:bool)
          n56 = case shown="True" w38 {
            tunnel: w26 -> [w110 w171]
            frame False {
              n57 = Unbundle By Name(w110) -> ("Motion Module.Rot Ver"=w140:refnum<vi>)
              n58 = Unbundle By Name(w110) -> ("Motion Module.Traction"=w145:refnum<vi>)
              n59 = property class="Bool (strict)"(reference=w145) -> (reference out=w143:refnum<vi>, error out=w144:errorcluster, "Value"=w147:bool)  [unwired: 1 in]
              n60 = property class="Bool (strict)"(reference=w140) -> (reference out=w142:refnum<vi>, error out=w141:errorcluster, "Value"=w146:bool)  [unwired: 1 in]
              n61 = Close Reference(reference=w143, error in (no error)=w144) -> ()  [unwired: 1 out]
              n62 = Close Reference(reference=w142, error in (no error)=w141) -> ()  [unwired: 1 out]
              n63 = Or(x=w146, y=w147) -> (x .or. y?=w131:bool)
              n64 = Unbundle By Name(w110) -> ("Loading Com Port.FFx(N)"=w137:refnum<vi>)
              n65 = Unbundle By Name(w110) -> ("Loading Com Port.FFy(N)"=w134:refnum<vi>)
              n66 = property class="Arr (strict)"(reference=w134) -> (reference out=w136:refnum<vi>, error out=w135:errorcluster, "Value"=w132:dbl[])  [unwired: 1 in]
              n67 = property class="Arr (strict)"(reference=w137) -> (reference out=w139:refnum<vi>, error out=w138:errorcluster, "Value"=w133:dbl[])  [unwired: 1 in]
              n68 = Close Reference(reference=w136, error in (no error)=w135) -> ()  [unwired: 1 out]
              n69 = Unbundle By Name(w110) -> ("Main Screen.zFF"=w129:refnum<vi>)
              n70 = Close Reference(reference=w139, error in (no error)=w138) -> ()  [unwired: 1 out]
              n71 = Select(t=w133, s=w131, f=w132) -> (s? t:f=w130:dbl[])
              n72 = property class="Bool (strict)"(reference=w129) -> (reference out=w127:refnum<vi>, error out=w128:errorcluster, "Value"=w126:bool)  [unwired: 1 in]
              n73 = call-poly <vilib>:"Mean.vi"("X"=w130) -> ("mean"=w118:dbl)  [unwired: 1 out]
              n74 = Close Reference(reference=w127, error in (no error)=w128) -> ()  [unwired: 1 out]
              n75 = Unbundle By Name(w110) -> ("Config Parameters.SAMPLES"=w117:refnum<vi>)
              n76 = Unbundle By Name(w110) -> ("Config Parameters.Re-initilaize"=w119:refnum<vi>)
              n77 = Unbundle By Name(w110) -> ("Config Parameters.Filter ON/OFF"=w125:refnum<vi>)
              n78 = case shown="True" w126 {
                tunnel: w110 -> [_ w162]
                tunnel: w118 -> [_ w160]
                frame False {
                }
                frame True {
                  n79 = Unbundle By Name(w162) -> ("Main Screen.zFF"=w163:refnum<vi>)
                  n80 = property class="Bool (strict)"(reference=w163, "Value"=FALSE) -> (reference out=w165:refnum<vi>, error out=w164:errorcluster)  [unwired: 1 in]
                  n81 = Close Reference(reference=w165, error in (no error)=w164) -> ()  [unwired: 1 out]
                  "Fload" <- w160
                }
              }
              n82 = local read "Fload"() -> (w106:dbl)
              n83 = Subtract(x=w118, y=w106) -> (x-y=w107:dbl)
              "Friction" <- w107
              n84 = property class="Bool (strict)"(reference=w125) -> (reference out=w123:refnum<vi>, error out=w124:errorcluster, "Value"=w122:bool)  [unwired: 1 in]
              n85 = property class="DigNum (strict)"(reference=w117) -> (reference out=w115:refnum<vi>, error out=w116:errorcluster, "Value"=w114:dbl)  [unwired: 1 in]
              n86 = property class="Bool (strict)"(reference=w119) -> (reference out=w121:refnum<vi>, error out=w120:errorcluster, "Value"=w108:bool)  [unwired: 1 in]
              n87 = Close Reference(reference=w123, error in (no error)=w124) -> ()  [unwired: 1 out]
              n88 = Close Reference(reference=w121, error in (no error)=w120) -> ()  [unwired: 1 out]
              n89 = Close Reference(reference=w115, error in (no error)=w116) -> ()  [unwired: 1 out]
              n90 = case shown="True" w122 {
                tunnel: w108 -> [_ w154]
                tunnel: w110 -> [_ w153]
                tunnel: w107 -> [w148 w152]
                tunnel: w114 -> [_ w151]
                tunnel: [w148 w150] -> w109
                tunnel: w108 -> [_ w149]
                frame False {
                }
                frame True {
                  n91 = case shown="True" w149 {
                    tunnel: w153 -> [_ w156]
                    frame False {
                    }
                    frame True {
                      n92 = Unbundle By Name(w156) -> ("Config Parameters.Re-initilaize"=w159:refnum<vi>)
                      n93 = property class="Bool (strict)"(reference=w159, "Value"=FALSE) -> (reference out=w157:refnum<vi>, error out=w158:errorcluster)  [unwired: 1 in]
                      n94 = Close Reference(reference=w157, error in (no error)=w158) -> ()  [unwired: 1 out]
                    }
                  }
                  n95 = call <vilib>:"Mean PtByPt.vi"("x"=w152, "sample length"=w151, "initialize"=w154) -> ("mean"=w150:dbl)  [unwired: 1 in, 1 out]
                }
              }
              n96 = Unbundle By Name(w110) -> ("Main Screen.Friction Force (N)"=w111:refnum<vi>)
              n97 = property class="DigNum (strict)"(reference=w111, "Value"=w109) -> (reference out=w113:refnum<vi>, error out=w112:errorcluster)  [unwired: 1 in]
              n98 = Close Reference(reference=w113, error in (no error)=w112) -> ()  [unwired: 1 out]
            }
            frame True {
              n99 = Unbundle By Name(w171) -> ("Loading Com Port.FORCE (N)"=w204:refnum<vi>)
              n100 = Unbundle By Name(w171) -> ("Loading Com Port.FFy(N)"=w183:refnum<vi>)
              n101 = property class="WFChart (strict)"(reference=w204) -> (reference out=w202:refnum<vi>, error out=w203:errorcluster, "History Data"=w168:dbl[][])  [unwired: 1 in]
              n102 = property class="Arr (strict)"(reference=w183) -> (reference out=w181:refnum<vi>, error out=w182:errorcluster, "Value"=w180:dbl[])  [unwired: 1 in]
              n103 = Unbundle By Name(w171) -> ("Main Screen.Friction Force (N)"=w192:refnum<vi>)
              n104 = Index Array(array=w168, index (col)=1 ("disabled index (col)")) -> (element=w167:dbl[])  [unwired: 1 in]
              n105 = Close Reference(reference=w202, error in (no error)=w203) -> ()  [unwired: 1 out]
              n106 = Close Reference(reference=w181, error in (no error)=w182) -> ()  [unwired: 1 out]
              n107 = Index Array(array=w180) -> (element=w174:dbl)  [unwired: 1 in]
              n108 = call-poly <vilib>:"Mean.vi"("X"=w167) -> ("mean"=w201:dbl)  [unwired: 1 out]
              n109 = Unbundle By Name(w171) -> ("Main Screen.CZ FF"=w179:refnum<vi>)
              n110 = Subtract(x=w167, y=w201) -> (x-y=w200:dbl[])
              n111 = property class="DigNum (strict)"(reference=w192) -> (reference out=w194:refnum<vi>, error out=w193:errorcluster, "Value"=w191:dbl)  [unwired: 1 in]
              n112 = property class="Bool (strict)"(reference=w179) -> (reference out=w177:refnum<vi>, error out=w178:errorcluster, "Value"=w176:bool)  [unwired: 1 in]
              n113 = call-poly <vilib>:"RMS.vi"("X"=w200) -> ("rms value"=w198:dbl)  [unwired: 1 out]
              n114 = Unbundle By Name(w171) -> ("Main Screen.zFF"=w190:refnum<vi>)
              n115 = Not A Number/Path/Refnum?(number/path/refnum=w198) -> (NaN/Path/Refnum?=w199:bool)
              n116 = Close Reference(reference=w194, error in (no error)=w193) -> ()  [unwired: 1 out]
              n117 = property class="Bool (strict)"(reference=w190) -> (reference out=w188:refnum<vi>, error out=w189:errorcluster, "Value"=w187:bool)  [unwired: 1 in]
              n118 = Close Reference(reference=w177, error in (no error)=w178) -> ()  [unwired: 1 out]
              n119 = Select(t=w191, s=w199, f=w198) -> (s? t:f=w186:dbl)
              n120 = case shown="True" w176 {
                tunnel: w171 -> [_ w207]
                tunnel: w174 -> [_ w205]
                frame False {
                }
                frame True {
                  n121 = Unbundle By Name(w207) -> ("Main Screen.CZ FF"=w208:refnum<vi>)
                  n122 = property class="Bool (strict)"(reference=w208, "Value"=FALSE) -> (reference out=w210:refnum<vi>, error out=w209:errorcluster)  [unwired: 1 in]
                  n123 = Close Reference(reference=w210, error in (no error)=w209) -> ()  [unwired: 1 out]
                  "Fload 3" <- w205
                }
              }
              n124 = Close Reference(reference=w188, error in (no error)=w189) -> ()  [unwired: 1 out]
              n125 = local read "Fload 2"() -> (w184:dbl)
              n126 = case shown="True" w187 {
                tunnel: w171 -> [_ w213]
                tunnel: w186 -> [_ w211]
                frame False {
                }
                frame True {
                  n127 = Unbundle By Name(w213) -> ("Main Screen.zFF"=w214:refnum<vi>)
                  n128 = property class="Bool (strict)"(reference=w214, "Value"=FALSE) -> (reference out=w216:refnum<vi>, error out=w215:errorcluster)  [unwired: 1 in]
                  n129 = Close Reference(reference=w216, error in (no error)=w215) -> ()  [unwired: 1 out]
                  "Fload 2" <- w211
                }
              }
              n130 = Unbundle By Name(w171) -> ("Main Screen.Friction Force (N)"=w195:refnum<vi>)
              n131 = local read "Fload 3"() -> (w175:dbl)
              n132 = Subtract(x=w186, y=w184) -> (x-y=w185:dbl)
              n133 = Subtract(x=w174, y=w175) -> (x-y=w169:dbl)
              n134 = property class="DigNum (strict)"(reference=w195, "Value"=w185) -> (reference out=w197:refnum<vi>, error out=w196:errorcluster)  [unwired: 1 in]
              n135 = Unbundle By Name(w171) -> ("Main Screen.Cyclic Friction Force (N)"=w172:refnum<vi>)
              n136 = Close Reference(reference=w197, error in (no error)=w196) -> ()  [unwired: 1 out]
              n137 = property class="DigNum (strict)"(reference=w172, "Value"=w169) -> (reference out=w170:refnum<vi>, error out=w173:errorcluster)  [unwired: 1 in]
              n138 = Close Reference(reference=w170, error in (no error)=w173) -> ()  [unwired: 1 out]
            }
          }
          n139 = call-poly <vilib>:"Mean.vi"("X"=w16) -> ("mean"=w78:dbl)  [unwired: 1 out]
          n140 = Negate(x=w78) -> (-x=w65:dbl)
          n141 = Unbundle By Name(w26) -> ("Main Screen.zNL 2"=w69:refnum<vi>)
          n142 = Unbundle By Name(w26) -> ("Motion Module.zNL"=w74:refnum<vi>)
          n143 = property class="Bool (strict)"(reference=w69) -> (reference out=w71:refnum<vi>, error out=w70:errorcluster, "Value"=w67:bool)  [unwired: 1 in]
          n144 = property class="Bool (strict)"(reference=w74) -> (reference out=w72:refnum<vi>, error out=w73:errorcluster, "Value"=w68:bool)  [unwired: 1 in]
          n145 = Close Reference(reference=w71, error in (no error)=w70) -> ()  [unwired: 1 out]
          n146 = Close Reference(reference=w72, error in (no error)=w73) -> ()  [unwired: 1 out]
          n147 = Or(x=w68, y=w67) -> (x .or. y?=w66:bool)
          n148 = case shown="True" w66 {
            tunnel: w65 -> [_ w240]
            tunnel: w26 -> [_ w233]
            frame False {
            }
            frame True {
              w232 = FALSE ("Value")
              n149 = Unbundle By Name(w233) -> ("Main Screen.zNL 2"=w234:refnum<vi>)
              n150 = Unbundle By Name(w233) -> ("Motion Module.zNL"=w239:refnum<vi>)
              n151 = property class="Bool (strict)"(reference=w234, "Value"=w232) -> (reference out=w236:refnum<vi>, error out=w235:errorcluster)  [unwired: 1 in]
              n152 = property class="Bool (strict)"(reference=w239, "Value"=w232) -> (reference out=w237:refnum<vi>, error out=w238:errorcluster)  [unwired: 1 in]
              n153 = Close Reference(reference=w236, error in (no error)=w235) -> ()  [unwired: 1 out]
              n154 = Close Reference(reference=w237, error in (no error)=w238) -> ()  [unwired: 1 out]
              "Zload" <- w240
            }
          }
          n155 = local read "Zload"() -> (w64:dbl)
          n156 = Subtract(x=w65, y=w64) -> (x-y=w59:dbl)
          n157 = Unbundle By Name(w26) -> ("PID.Vertical load (N)"=w77:refnum<vi>)
          n158 = Unbundle By Name(w26) -> ("Config Parameters.Apply Filter (Load)"=w61:refnum<vi>)
          n159 = property class="DigNum (strict)"(reference=w77, "Value"=w59) -> (reference out=w75:refnum<vi>, error out=w76:errorcluster)  [unwired: 1 in]
          n160 = property class="Bool (strict)"(reference=w61) -> (reference out=w63:refnum<vi>, error out=w62:errorcluster, "Value"=w60:bool)  [unwired: 1 in]
          n161 = Close Reference(reference=w75, error in (no error)=w76) -> ()  [unwired: 1 out]
          n162 = Close Reference(reference=w63, error in (no error)=w62) -> ()  [unwired: 1 out]
          n163 = case shown="True" w60 {
            tunnel: w26 -> [_ w228]
            tunnel: w59 -> [w217 w222]
            tunnel: [w217 w219] -> w56
            frame False {
            }
            frame True {
              n164 = Unbundle By Name(w228) -> ("Config Parameters.Filter%"=w231:refnum<vi>)
              n165 = property class="DigNum (strict)"(reference=w231) -> (reference out=w229:refnum<vi>, error out=w230:errorcluster, "Value"=w227:dbl)  [unwired: 1 in]
              n166 = Close Reference(reference=w229, error in (no error)=w230) -> ()  [unwired: 1 out]
              n167 = Multiply(x=w227, y=0.01) -> (x*y=w224:dbl)
              n168 = local read "Load Temp"() -> (w218:dbl)
              n169 = Subtract(x=1.0, y=w224) -> (x-y=w223:dbl)
              n170 = Multiply(x=w222, y=w223) -> (x*y=w221:dbl)
              n171 = Multiply(x=w224, y=w218) -> (x*y=w220:dbl)
              n172 = Add(x=w221, y=w220) -> (x+y=w219:dbl)
            }
          }
          n173 = Not A Number/Path/Refnum?(number/path/refnum=w56) -> (NaN/Path/Refnum?=w58:bool)
          n174 = Unbundle By Name(w26) -> ("Motion Module.NL disp"=w53:refnum<vi>)
          n175 = Unbundle By Name(w26) -> ("Main Screen.NL disp 2"=w52:refnum<vi>)
          n176 = Select(t=0.0, s=w58, f=w56) -> (s? t:f=w49:dbl)
          "Load Temp" <- w49
          n177 = property class="DigNum (strict)"(reference=w53, "Value"=w49) -> (reference out=w55:refnum<vi>, error out=w54:errorcluster)  [unwired: 1 in]
          n178 = property class="DigNum (strict)"(reference=w52, "Value"=w49) -> (reference out=w50:refnum<vi>, error out=w51:errorcluster)  [unwired: 1 in]
          n179 = Close Reference(reference=w55, error in (no error)=w54) -> ()  [unwired: 1 out]
          n180 = Close Reference(reference=w50, error in (no error)=w51) -> ()  [unwired: 1 out]
        }
      }
    }
    frame Error {
    }
  }
  "error out" <- w1
